vi "numCmd_Send_TwoDbl.vi"(7 "Command Name":string, 10 "Value 2":dbl, 11 "Value 1":dbl) -> (0 "error out":errorcluster)   [LabVIEW 2019, in "Trajectory_Library.lvlib"]
uses:
  Trajectory_Library.lvlib
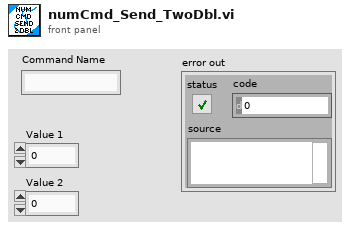
[diagram p1: front panel]
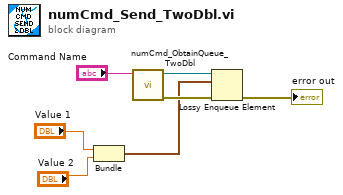
[diagram p0: block diagram]
diagram:
  n1 = Bundle("Value 1"="Value 1", "Value 2"="Value 2") -> (w2:cluster{"Value 1":dbl, "Value 2":dbl})  [unwired: 1 in]
  n2 = call "numCmd_ObtainQueue_TwoDbl.vi"("Command Name"="Command Name") -> ("error out"=w4:errorcluster, "queue out"=w5:refnum<queue>)  [unwired: 9 in]
  n3 = Lossy Enqueue Element(queue=w5, element=w2, error in (no error)=w4) -> (error out=→"error out":errorcluster)  [unwired: 3 out]
